vi "Configure List Step Radio Band.vi"(8 "error in (no error)":errorcluster {"code" format="%.0x"}, 9 "RadioBand (I Agxs An 5ss List Sequencer Setup Radio Band None)":i32(ring) items=["I Agxs An 5ss List Sequencer Setup Radio Band None"=0, "I Agxs An 5ss List Sequencer Setup Radio Bandpgsm"=1, "I Agxs An 5ss List Sequencer Setup Radio Bandegsm"=2, "I Agxs An 5ss List Sequencer Setup Radio Bandrgsm"=3, "I Agxs An 5ss List Sequencer Setup Radio Banddcs1800"=4, "I Agxs An 5ss List Sequencer Setup Radio Bandpcs1900"=5, "I Agxs An 5ss List Sequencer Setup Radio Bandtgsm810"=6, "I Agxs An 5ss List Sequencer Setup Radio Bandgsm450"=7, "I Agxs An 5ss List Sequencer Setup Radio Bandgsm480"=8, "I Agxs An 5ss List Sequencer Setup Radio Bandgsm700"=9, "I Agxs An 5ss List Sequencer Setup Radio Bandgsm850"=10, "I Agxs An 5ss List Sequencer Setup Radio Bandbandi"=11, "I Agxs An 5ss List Sequencer Setup Radio Bandbandii"=12, "I Agxs An 5ss List Sequencer Setup Radio Bandbandiii"=13, "I Agxs An 5ss List Sequencer Setup Radio Bandbandiv"=14, "I Agxs An 5ss List Sequencer Setup Radio Bandbandv"=15, "I Agxs An 5ss List Sequencer Setup Radio Bandbandvi"=16, "I Agxs An 5ss List Sequencer Setup Radio Bandbandvii"=17, "I Agxs An 5ss List Sequencer Setup Radio Bandbandviii"=18, "I Agxs An 5ss List Sequencer Setup Radio Bandbandix"=19, "I Agxs An 5ss List Sequencer Setup Radio Bandbandx"=20, "I Agxs An 5ss List Sequencer Setup Radio Bandbandxi"=21, "I Agxs An 5ss List Sequencer Setup Radio Bandbandxii"=22, "I Agxs An 5ss List Sequencer Setup Radio Bandbandxiii"=23, "I Agxs An 5ss List Sequencer Setup Radio Bandbandxiv"=24, "I Agxs An 5ss List Sequencer Setup Radio Bandbandxix"=25, "I Agxs An 5ss List Sequencer Setup Radio Banduscell"=26, "I Agxs An 5ss List Sequencer Setup Radio Banduspcs"=27, "I Agxs An 5ss List Sequencer Setup Radio Bandjapan"=28, "I Agxs An 5ss List Sequencer Setup Radio Bandkorean"=29, "I Agxs An 5ss List Sequencer Setup Radio Bandnmt"=30, "I Agxs An 5ss List Sequencer Setup Radio Bandimt 2k"=31, "I Agxs An 5ss List Sequencer Setup Radio Bandupper"=32, "I Agxs An 5ss List Sequencer Setup Radio Bandsecond"=33, "I Agxs An 5ss List Sequencer Setup Radio Bandpamr400"=34, "I Agxs An 5ss List Sequencer Setup Radio Bandpamr800"=35, "I Agxs An 5ss List Sequencer Setup Radio Bandimtext"=36, "I Agxs An 5ss List Sequencer Setup Radio Bandpcs 1dot 9g"=37, "I Agxs An 5ss List Sequencer Setup Radio Bandaws"=38, "I Agxs An 5ss List Sequencer Setup Radio Bandus 2dot 5g"=39, "I Agxs An 5ss List Sequencer Setup Radio Bandpublic"=40, "I Agxs An 5ss List Sequencer Setup Radio Bandlower"=41, "I Agxs An 5ss List Sequencer Setup Radio Bandband1"=42, "I Agxs An 5ss List Sequencer Setup Radio Bandband2"=43, "I Agxs An 5ss List Sequencer Setup Radio Bandband3"=44, "I Agxs An 5ss List Sequencer Setup Radio Bandband4, I Agxs An 5ss List Sequencer Setup Radio Bandband9"=45, "I Agxs An 5ss List Sequencer Setup Radio Bandband5"=46, "I Agxs An 5ss List Sequencer Setup Radio Bandband6"=47, "I Agxs An 5ss List Sequencer Setup Radio Bandband7"=48, "I Agxs An 5ss List Sequencer Setup Radio Bandband8"=49, "I Agxs An 5ss List Sequencer Setup Radio Bandbanda"=87, "I Agxs An 5ss List Sequencer Setup Radio Bandband10"=50, "I Agxs An 5ss List Sequencer Setup Radio Bandband11"=51, "I Agxs An 5ss List Sequencer Setup Radio Bandband12"=52, "I Agxs An 5ss List Sequencer Setup Radio Bandband13"=53, "I Agxs An 5ss List Sequencer Setup Radio Bandband14"=54, "I Agxs An 5ss List Sequencer Setup Radio Bandbandb"=88, "I Agxs An 5ss List Sequencer Setup Radio Bandbandc"=89, "I Agxs An 5ss List Sequencer Setup Radio Bandband17"=55, "I Agxs An 5ss List Sequencer Setup Radio Bandband18"=56, "I Agxs An 5ss List Sequencer Setup Radio Bandband19"=57, "I Agxs An 5ss List Sequencer Setup Radio Bandband20"=58, "I Agxs An 5ss List Sequencer Setup Radio Bandband21"=59, "I Agxs An 5ss List Sequencer Setup Radio Bandbandd"=90, "I Agxs An 5ss List Sequencer Setup Radio Bandbande"=91, "I Agxs An 5ss List Sequencer Setup Radio Bandband24"=60, "I Agxs An 5ss List Sequencer Setup Radio Bandband25"=61, "I Agxs An 5ss List Sequencer Setup Radio Bandband26"=62, "I Agxs An 5ss List Sequencer Setup Radio Bandband27"=63, "I Agxs An 5ss List Sequencer Setup Radio Bandband28"=64, "I Agxs An 5ss List Sequencer Setup Radio Bandband29"=65, "I Agxs An 5ss List Sequencer Setup Radio Bandband30"=66, "I Agxs An 5ss List Sequencer Setup Radio Bandband31"=67, "I Agxs An 5ss List Sequencer Setup Radio Bandband65"=68, "I Agxs An 5ss List Sequencer Setup Radio Bandband66"=69, "I Agxs An 5ss List Sequencer Setup Radio Bandband68"=70, "I Agxs An 5ss List Sequencer Setup Radio Bandband252"=71, "I Agxs An 5ss List Sequencer Setup Radio Bandband255"=72, "I Agxs An 5ss List Sequencer Setup Radio Bandband33"=73, "I Agxs An 5ss List Sequencer Setup Radio Bandband34"=74, "I Agxs An 5ss List Sequencer Setup Radio Bandband35"=75, "I Agxs An 5ss List Sequencer Setup Radio Bandband36"=76, "I Agxs An 5ss List Sequencer Setup Radio Bandband37"=77, "I Agxs An 5ss List Sequencer Setup Radio Bandband38"=78, "I Agxs An 5ss List Sequencer Setup Radio Bandband39"=79, "I Agxs An 5ss List Sequencer Setup Radio Bandband40"=80, "I Agxs An 5ss List Sequencer Setup Radio Bandband41"=81, "I Agxs An 5ss List Sequencer Setup Radio Bandband42"=82, "I Agxs An 5ss List Sequencer Setup Radio Bandband43"=83, "I Agxs An 5ss List Sequencer Setup Radio Bandband44"=84, "I Agxs An 5ss List Sequencer Setup Radio Bandband45"=85, "I Agxs An 5ss List Sequencer Setup Radio Bandband46"=86, "I Agxs An 5ss List Sequencer Setup Radio Bandbandf"=92], 10 "StepIndex":i32 format="%.0g", 11 "instrument handle":refnum<k15>) -> (0 "error out":errorcluster {"code" format="%.0x"}, 3 "instrument handle out":refnum<k15>)   [LabVIEW 2009, in "Keysight XSAn.lvlib"]
doc: "Configure radio band standard of the selected step.\n\nSupported Models: M8920A, M9420A, M9421A."
uses:
  <instrlib>/Keysight XSAn/Keysight XSAn.lvlib
  AgXSAn.dll
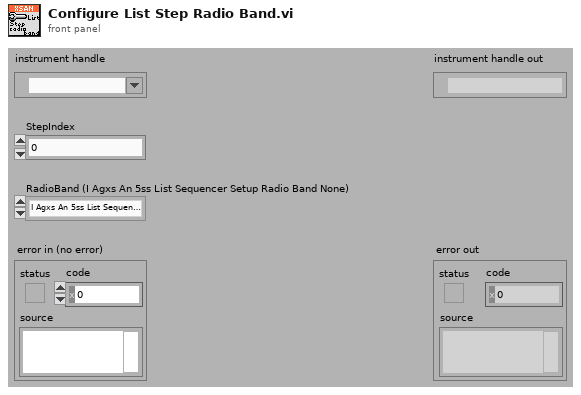
[diagram p1: front panel]
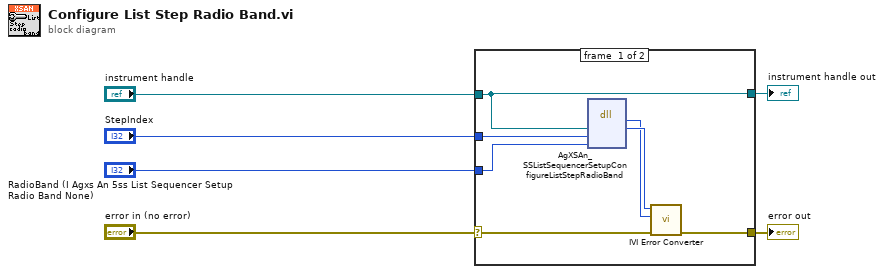
[diagram p0: block diagram]
diagram:
  n1 = case shown="No Error" "error in (no error)" {
    selector: "error in (no error)" -> [w11 w15]
    tunnel: [w10 w15] -> w6
    tunnel: "instrument handle" -> [w7 w14]
    tunnel: "StepIndex" -> [w9 _]
    tunnel: "RadioBand (I Agxs An 5ss List Sequencer Setup Radio Band None)" -> [w8 _]
    tunnel: [w7 w14] -> w1
    frame #0 {
      n2 = dll-call lib="AgXSAn**.dll" fn="AgXSAn_SSListSequencerSetupConfigureListStepRadioBand"("Vi"=w7, "StepIndex"=w9, "RadioBand"=w8) -> (w12:i32, "Vi"=w13:u32)  [unwired: 5 in, 2 out]
      n3 = call <instrlib>:"IVI Error Converter.vi"("error in (no error)"=w11, "IVI error code (0)"=w12, "instrument handle"=w13) -> ("error out"=w10:errorcluster)  [unwired: 7 in, 1 out]
    }
    frame #1 {
    }
  }
  "error out" <- w6
  "instrument handle out" <- w1
